vi "Best Focus.vi"(6 "Component":T1, 8 "error in (no error)":errorcluster, 9 "Inc by":dbl=-0.1 format="%#_13g", 11 "Gantry In":refnum<k24>) -> (0 "error out":errorcluster, 1 "Error?":bool, 2 "max value":dbl, 3 "Gantry Out":refnum<k24>)   [LabVIEW 2021, in "Component Tray.lvclass"]
uses:
  Component Tray.lvclass
  C:/Program Files (x86)/Aerotech/A3200/LabVIEW/2010/Bin/Aerotech.A3200.dll
  Program Files (x86)/Aerotech/A3200/LabVIEW/2010/Bin/Aerotech.A3200.dll
  Find Component.ctl
  Controller/Camera/Machine Vision.ctl
  Component Tray.lvclass/Component Tray.ctl
  Controller/Motion/A3200/A3200.lvclass
  Controller/Camera/Camera.lvclass
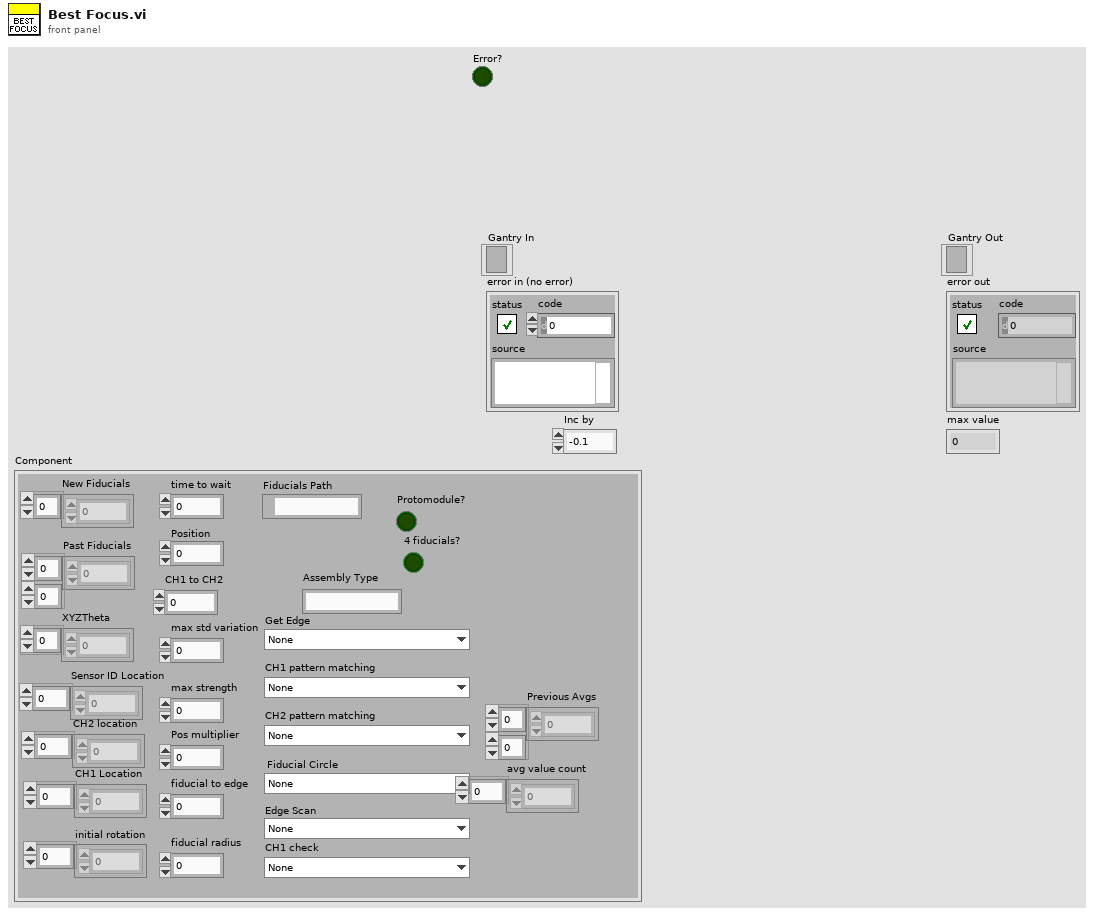
[diagram p1: front panel]
types:
  T1 = typedef "Component Tray.lvclass/Find Component.ctl" = cluster{"New Fiducials":dbl[], "Past Fiducials":dbl[][], "XYZTheta":dbl[], "Fiducials Path":path, "Position":i32, "CH1 Location":dbl[], "Sensor ID Location":dbl[], "initial rotation":dbl[], "CH2 location":dbl[], "max std variation":dbl, "max strength":dbl, "CH2 pattern matching":T2, "Fiducial Circle":T2, "Get Edge":T2, "Pos multiplier":dbl, "time to wait":u32, "fiducial to edge":dbl, "Protomodule?":bool, "Assembly Type":string, "CH1 to CH2":dbl, "Tray Number":string, "fiducial radius":dbl, "4 fiducials?":bool, "CH1 check":T2, "Edge Scan":T2, "CH1 pattern matching":T2, "Sensor Thickness":dbl, "Previous Avgs":dbl[][], "avg value count":dbl[]}
  T2 = typedef "Camera.lvclass/Machine Vision.ctl" = enum16{"None", "Assembly Tray Circle", "Assembly Tray Fiducial", "Partial Hexaboard", "sensor edge init", "HB edge init", "sensor edge pos1", "sensor edge pos2", "HB edge pos1", "HB edge pos2", "Sensor CH1-2", "HB CH1", "HB CH2", "V3 Sensor Circle", "Hexaboard Circle", "sensor CH1 check", "HB CH1 check ", "sensor ID"}
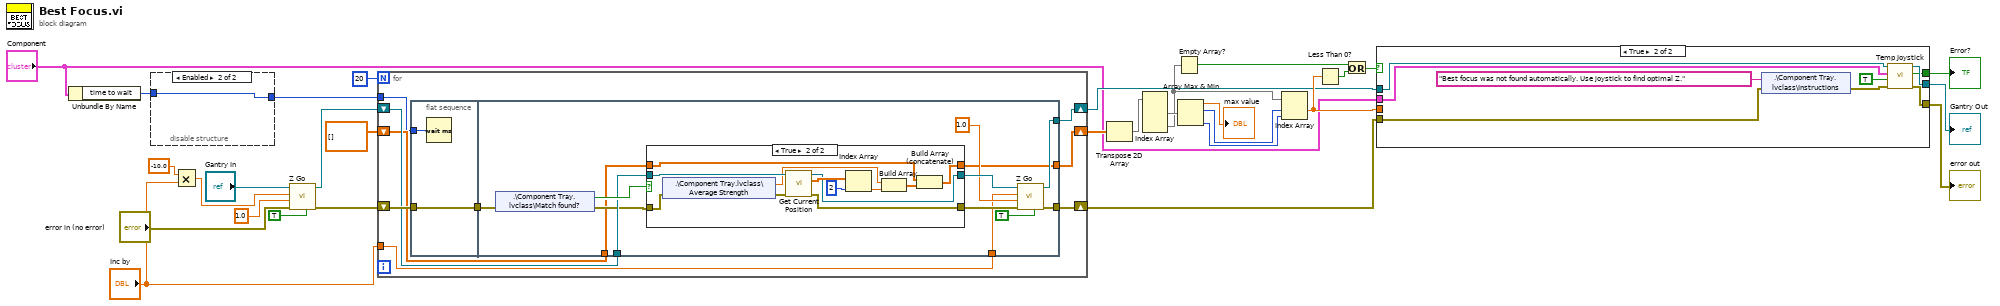
[diagram p0: block diagram]
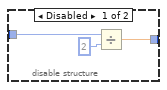
[diagram p2: hidden frame]
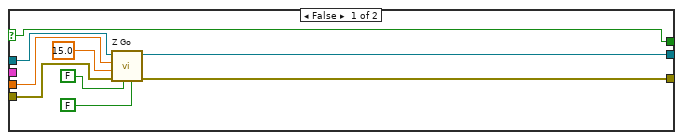
[diagram p3: hidden frame]
diagram:
  n1 = Unbundle By Name("Component") -> ("time to wait"=w6:u32)
  n2 = disable-structure shown="Enabled" {
    disable-tunnel: w6 -> [w33 w34]
    disable-tunnel: [w31 w34] -> w5
    frame Disabled {
      n3 = Divide(x=w33, y=u32 2) -> (x/y=w31:dbl)
    }
    frame Enabled {
    }
  }
  n4 = Multiply(x=-10.0, y="Inc by") -> (x*y=w3:dbl)
  n5 = call "Z Go.vi"("Increment"=TRUE, "error in (no error)"="error in (no error)", "Speed In"=1.0, "Position In"=w3, "Gantry In"="Gantry In") -> ("error out"=w28:errorcluster, "Gantry Out"=w27:refnum<k24>)  [unwired: 3 in, 2 out]
  n6 = for {
    N: 20 -> [_]
    shift-right: [w39] -> w17
    shift-left: w28 -> [w43]
    shift-right: [w40] -> w15
    shift-left: w27 -> [w41]
    shift-right: [w38] -> w23
    shift-left: dbl[][] [] -> [w37]
    tunnel: w5 -> [w36]
    tunnel: "Inc by" -> [w35]
    n7 = flat-sequence {
      tunnel: w43 -> [w45]
      tunnel: [w45] -> w42
      tunnel: w36 -> [w44]
      tunnel: w41 -> [w56]
      tunnel: w42 -> [w57]
      tunnel: [w52] -> w40
      tunnel: [w51] -> w39
      tunnel: [w48] -> w38
      tunnel: w37 -> [w47]
      tunnel: w35 -> [w46]
      frame #0 {
        n8 = Wait (ms)(milliseconds to wait=w44) -> ()  [unwired: 1 out]
      }
      frame #1 {
        n9 = shared-variable ".\\Component Tray.lvclass\\Match found?"(error in=w57) -> (w58:bool, error out=w55:errorcluster)
        n10 = case shown="True" w58 {
          tunnel: w56 -> [w61 w73]
          tunnel: w55 -> [w60 w71]
          tunnel: [w61 w66] -> w54
          tunnel: [w60 w65] -> w53
          tunnel: [w59 w63] -> w48
          tunnel: w47 -> [w59 w62]
          frame False {
          }
          frame True {
            n11 = shared-variable ".\\Component Tray.lvclass\\Average Strength"(error in=w71) -> (w67:dbl, error out=w72:errorcluster)
            n12 = call "Get Current Position.vi"("error in (no error)"=w72, "Gantry In"=w73) -> ("error out"=w65:errorcluster, "XYZTheta Out"=w70:dbl[], "Gantry Out"=w66:refnum<k24>)  [unwired: 7 in]
            n13 = Index Array(array=w70, index=2) -> (element=w68:dbl)
            n14 = Build Array(w67, w68) -> (w64:dbl[])
            n15 = Build Array (concatenate)(w62, w64) -> (w63:dbl[][])
          }
        }
        n16 = call "Z Go.vi"("Increment"=TRUE, "error in (no error)"=w53, "Speed In"=1.0, "Position In"=w46, "Gantry In"=w54) -> ("error out"=w51:errorcluster, "Gantry Out"=w52:refnum<k24>)  [unwired: 3 in, 2 out]
      }
    }
  }
  n17 = Transpose 2D Array(2D array=w23) -> (transposed array=w26:dbl[][])
  n18 = Index Array(array=w26) -> (element #1=w24:dbl[], element #2=w12:dbl[])  [unwired: 4 in]
  n19 = Empty Array?(array=w12) -> (empty?=w11:bool)
  n20 = Array Max & Min(array=w24) -> (max value=→"max value":dbl, max index (indices)=w25:i32, min index (indices)=w18:i32)  [unwired: 1 out]
  n21 = Index Array(array=w12, index #1=w25, index #2=w18) -> (element #1=w16:dbl)  [unwired: 1 out]
  n22 = Less Than 0?(x=w16) -> (x < 0?=w10:bool)
  n23 = Or(x=w11, y=w10) -> (x .or. y?=w9:bool)
  n24 = case shown="True" w9 {
    selector: w9 -> [w74 _]
    tunnel: w17 -> [w82 w87]
    tunnel: w16 -> [w81 _]
    tunnel: w15 -> [w80 w91]
    tunnel: [w79 w89] -> w14
    tunnel: [w78 w90] -> w13
    tunnel: [w74 w84] -> w8
    tunnel: "Component" -> [_ w83]
    frame False {
      n25 = call "Z Go.vi"("Increment"=FALSE, "Return Immediately"=FALSE ("Increment"), "error in (no error)"=w82, "Speed In"=15.0 ("Speed"), "Position In"=w81, "Gantry In"=w80) -> ("error out"=w79:errorcluster, "Gantry Out"=w78:refnum<k24>)  [unwired: 2 in, 2 out]
    }
    frame True {
      n26 = shared-variable ".\\Component Tray.lvclass\\Instructions"("Best focus was not found automatically. Use joystick to find optimal Z." ("Instructions"), error in=w87) -> (error out=w86:errorcluster)
      n27 = call "Temp Joystick.vi"("error in (no error)"=w86, "Fiducial?"=TRUE, "Component"=w83, "Gantry In"=w91) -> ("error out"=w89:errorcluster, "Error?"=w84:bool, "Gantry Out"=w90:refnum<k24>)  [unwired: 5 in]
    }
  }
  "Gantry Out" <- w13
  "error out" <- w14
  "Error?" <- w8
